vi "meta_openMetaFile.vi"(8 "error in":errorcluster, 11 "path":path) -> (0 "error out":errorcluster, 3 "meta file":T1)   [LabVIEW 2017, in "NI_ExcelFile.lvlib"]
uses:
  <vilib>/express/express shared/NI_ExcelFile/NI_ExcelFile.lvlib
  <vilib>/express/express shared/NI_ExcelFile/Ctrls/meta_file.ctl
  <vilib>/express/express shared/NI_ExcelFile/Ctrls/meta_Block.ctl
  <vilib>/express/express shared/NI_ExcelFile/Ctrls/meta_BlockType.ctl
  <vilib>/express/express shared/NI_ExcelFile/Ctrls/NITag.ctl
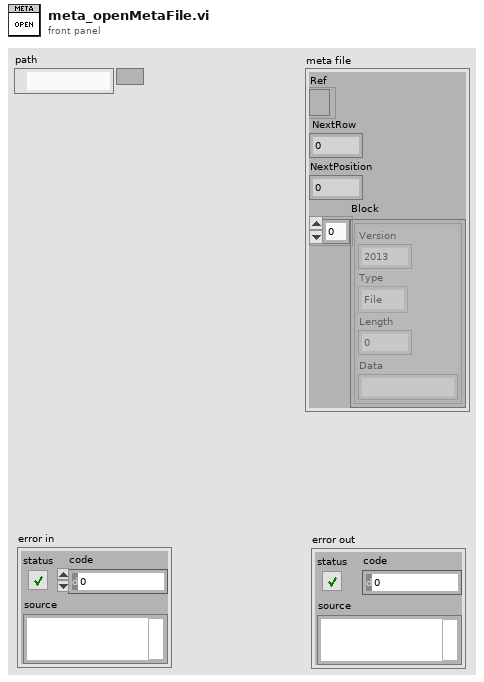
[diagram p1: front panel]
types:
  T1 = typedef "NI_ExcelFile.lvlib/meta_file.ctl" = cluster{"Ref":refnum<file>, "NextRow":i32, "NextPosition":i64, "Block":T2[]}
  T2 = typedef "NI_ExcelFile.lvlib/meta_Block.ctl" = cluster{"Version":u16, "Type":T3, "Length":i32, "Data":string}
  T3 = typedef "NI_ExcelFile.lvlib/meta_BlockType.ctl" = enum16{"NITag", "File", "Column"}
  T4 = typedef "NI_ExcelFile.lvlib/NITag.ctl" = string
  T5 = enum16{"open", "replace", "create", "open or create", "replace or create", "replace or create with confirmation"}
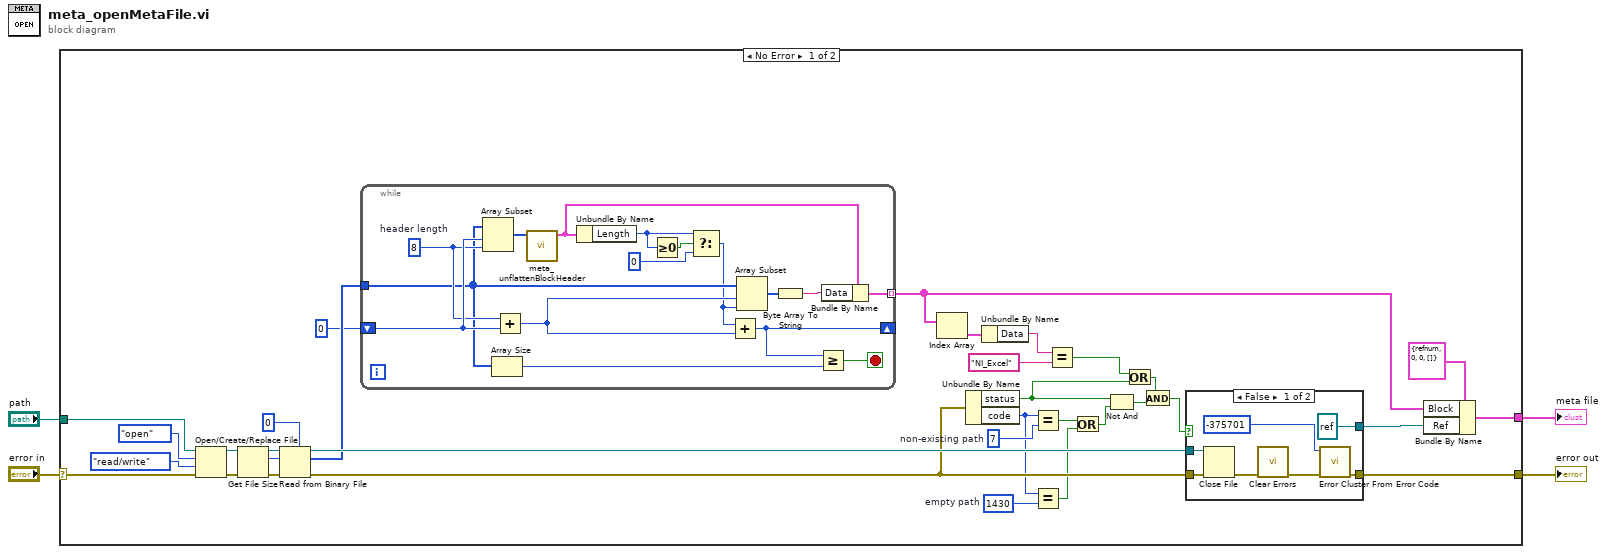
[diagram p0: block diagram]
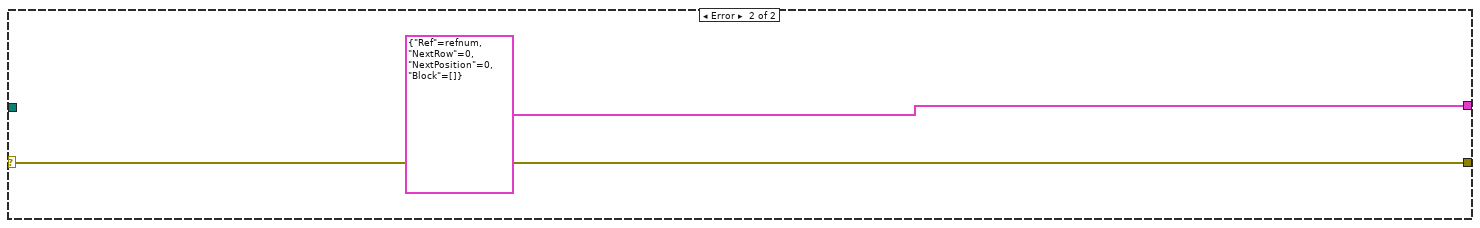
[diagram p3: hidden frame]
diagram:
  n1 = case shown="No Error" "error in" {
    selector: "error in" -> [w33 w64]
    tunnel: [w30 T1 {"Ref"=refnum, "NextRow"=0, "NextPosition"=0, "Block"=[]} ("meta file")] -> w4
    tunnel: [w32 w64] -> w3
    tunnel: "path" -> [w34 _]
    frame No Error {
      w8 = 1430  # empty path
      w16 = 7  # non-existing path
      n2 = Open/Create/Replace File(file path (use dialog)=w34, error in=w33, operation (0:open)=T5."open", access (0:read/write)=enum16{"read/write", "read-only", "write-only"}."read/write") -> (refnum out=w24:refnum<file>, error out=w25:errorcluster)  [unwired: 2 in, 1 out]
      n3 = Get File Size(file=w24, error in=w25) -> (refnum out=w28:refnum<file>, size (in bytes)=w27:i64, 0:w29:errorcluster)
      n4 = Read from Binary File(5:u8 0, 8:w29, 10:w27, 11:w28) -> (0:w17:errorcluster, 2:w22:u8[], 3:w23:refnum<file>)  [unwired: 2 in, 1 out]
      n5 = while {
        tunnel: w22 -> [w45]
        shift-right: [w44] -> _
        shift-left: 0 -> [w52]
        tunnel: [w47] -> w12 mode=indexing
        stop <- w42 stop-if-true
        w51 = 8  # header length
        n6 = Array Subset(array=w45, index=w52, length=w51) -> (w53:u8[])
        n7 = Array Size(array=w45) -> (size(s)=w43:i32)
        n8 = Add(x=w51, y=w52) -> (x+y=w46:i32)
        n9 = call <vilib>:"meta_unflattenBlockHeader.vi"("block header data"=w53) -> ("block out"=w49:T2)  [unwired: 10 in]
        n10 = Unbundle By Name(w49) -> ("Length"=w39:i32)
        n11 = Greater Or Equal To 0?(x=w39) -> (x >= 0?=w40:bool)
        n12 = Select(t=w39, s=w40, f=0) -> (s? t:f=w41:i32)
        n13 = Add(x=w41, y=w46) -> (x+y=w44:i32)
        n14 = Array Subset(array=w45, index=w46, length=w41) -> (w50:u8[])
        n15 = Byte Array To String(unsigned byte array=w50) -> (string=w48:string)
        n16 = Greater Or Equal?(x=w44, y=w43) -> (x >= y?=w42:bool)
        n17 = Bundle By Name(cluster=w49, "Data"=w48) -> (w47:T2)
      }
      n18 = Index Array(array=w12) -> (element=w20:T2)  [unwired: 1 in]
      n19 = Unbundle By Name(w17) -> ("status"=w10:bool, "code"=w9:i32)
      n20 = Unbundle By Name(w20) -> ("Data"=w19:string)
      n21 = Equal?(x=w9, y=w16) -> (x = y?=w7:bool)
      n22 = Equal?(x=w9, y=w8) -> (x = y?=w6:bool)
      n23 = Equal?(x=w19, y=T4 "NI_Excel" ("NITag")) -> (x = y?=w15:bool)
      n24 = Or(x=w7, y=w6) -> (x .or. y?=w5:bool)
      n25 = Not And(1:w5, 2:w10) -> (0:w14:bool)
      n26 = Or(x=w15, y=w10) -> (x .or. y?=w11:bool)
      n27 = And(x=w11, y=w14) -> (x .and. y?=w13:bool)
      n28 = case shown="False" w13 {
        tunnel: [w57 w62] -> w32
        tunnel: w17 -> [w60 w62]
        tunnel: [refnum<file> refnum ("refnum out") w61] -> w31
        tunnel: w23 -> [w59 w61]
        frame False {
          n29 = Close File(refnum=w59, error in=w60) -> (error out=w56:errorcluster)  [unwired: 1 out]
          n30 = call <vilib>:"Clear Errors.vi"("error in (no error)"=w56) -> ("error out"=w54:errorcluster)  [unwired: 5 in, 1 out]
          n31 = call <vilib>:"Error Cluster From Error Code.vi"("error in (no error)"=w54, "error code (0)"=-375701) -> ("error out"=w57:errorcluster)  [unwired: 7 in]
        }
        frame True {
        }
      }
      n32 = Bundle By Name(cluster=T1 {"Ref"=refnum, "NextRow"=0, "NextPosition"=0, "Block"=[]} ("meta file"), "Block"=w12, "Ref"=w31) -> (w30:T1)
    }
    frame Error {
    }
  }
  "meta file" <- w4
  "error out" <- w3
